vi "New Event Input.vi"(8 "error in (no error)":errorcluster, 11 "Descriptor":string) -> (0 "error out":errorcluster, 3 "event_input out":refnum<class "Event Input.lvclass">)   [LabVIEW 2015, in "Event Input.lvclass"]
uses:
  Event Input.lvclass
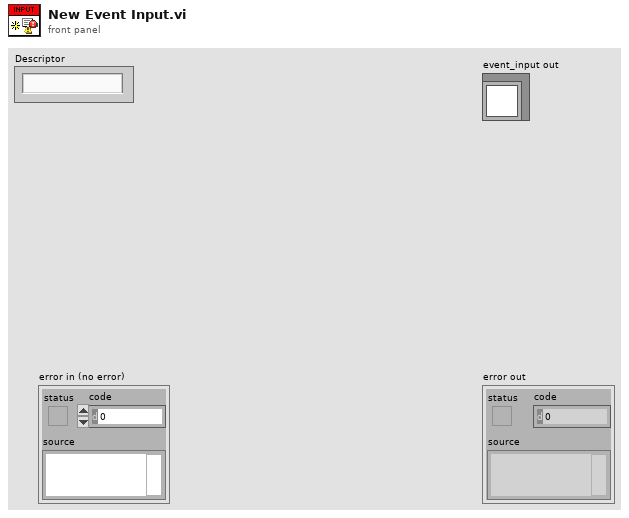
[diagram p1: front panel]
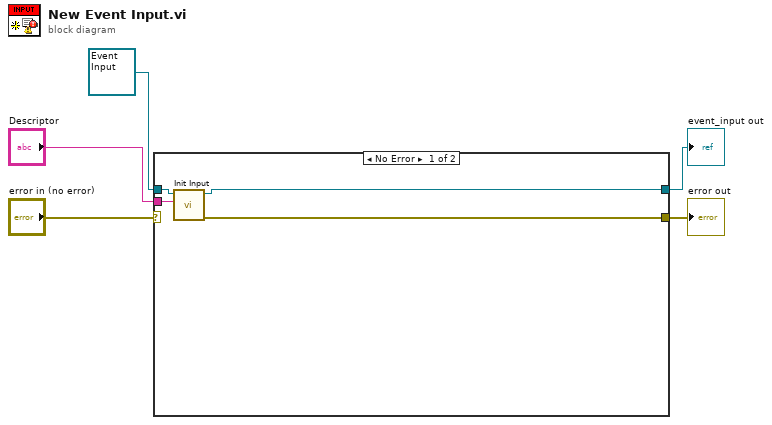
[diagram p0: block diagram]
diagram:
  n1 = case shown="No Error" "error in (no error)" {
    selector: "error in (no error)" -> [_ w11]
    tunnel: [w7 w11] -> w4
    tunnel: [w6 w10] -> w2
    tunnel: refnum<class "Event Input.lvclass"> refnum ("event_input in") -> [w9 w10]
    tunnel: "Descriptor" -> [w8 _]
    frame No Error {
      n2 = call-dynamic "Init Input.vi"("Descriptor"=w8, "input in"=w9) -> ("error out"=w7:errorcluster, "input out"=w6:refnum<class "Event Input.lvclass">)  [unwired: 8 in]
    }
    frame Error {
    }
  }
  "error out" <- w4
  "event_input out" <- w2
